vi "Faults_To_String_Array.vi"(0 "Write Header ?":bool, 1 "Fault Table Entry":T1[](array[typedef]), 5 "Error In":errorcluster) -> (15 "Fault Header String Array":string[](array[string]), 16 "Fault ERD Number String Array":string[](array[string]), 17 "Fault Data String Array":string[](array[string]), 19 "Error Out":errorcluster)   [LabVIEW 2023]
uses:
  type defs/Fault_Table_Info.ctl
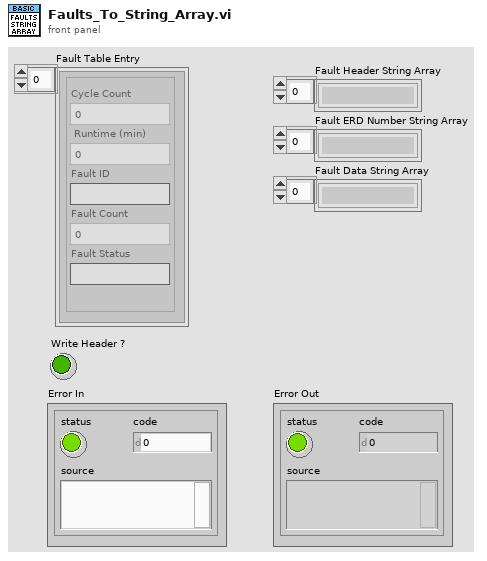
[diagram p1: front panel]
types:
  T1 = typedef "Fault_Table_Info.ctl" = cluster{"Cycle Count":u32, " Runtime (min) ":u32, "Fault Status":string, "Fault ID":string, "Fault Count":u16}
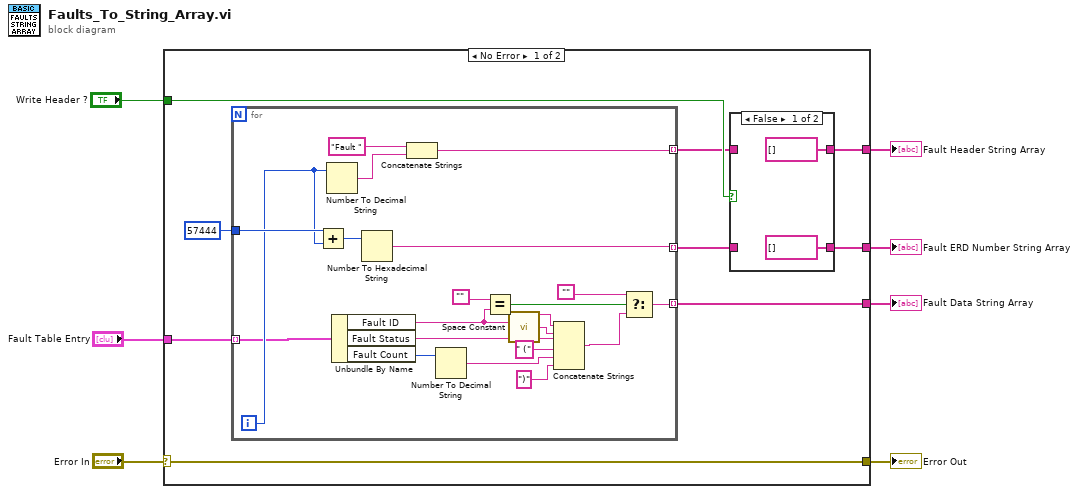
[diagram p0: block diagram]
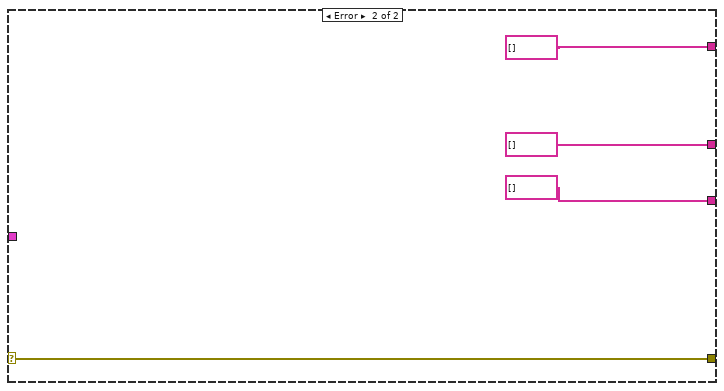
[diagram p3: hidden frame]
diagram:
  n1 = case shown="No Error" "Error In" {
    selector: "Error In" -> [w14 w43]
    tunnel: "Fault Table Entry" -> [w16 _]
    tunnel: [w15 string[] []] -> w6
    tunnel: [w14 w43] -> w4
    tunnel: [w10 string[] []] -> w3
    tunnel: [w8 string[] []] -> w2
    tunnel: "Write Header ?" -> [w12 _]
    frame No Error {
      n2 = for {
        tunnel: [w33] -> w15 mode=indexing
        tunnel: w16 -> [w27] mode=indexing
        tunnel: [w31] -> w11 mode=indexing
        tunnel: 57444 -> [w30]
        tunnel: [w28] -> w9 mode=indexing
        i -> [w29]
        n3 = Add(x=w30, y=w29) -> (x+y=w21:i32)
        n4 = Number To Decimal String(number=w29) -> (decimal integer string=w22:string)  [unwired: 1 in]
        n5 = Unbundle By Name(w27) -> ("Fault ID"=w26:string, "Fault Status"=w25:string, "Fault Count"=w24:u16)
        n6 = Number To Hexadecimal String(2:w21) -> (0:w28:string)  [unwired: 1 in]
        n7 = Concatenate Strings("Fault ", w22) -> (w31:string)
        n8 = Number To Decimal String(number=w24) -> (decimal integer string=w38:string)  [unwired: 1 in]
        n9 = Equal?(x="", y=w26) -> (x = y?=w35:bool)
        n10 = call <vilib>:"Space Constant.vi"() -> ("String"=w40:string)
        n11 = Concatenate Strings(w26, w40, w25, " (" ("string"), w38, ")" ("string")) -> (w34:string)
        n12 = Select(t="", s=w35, f=w34) -> (s? t:f=w33:string)
      }
      n13 = case shown="False" w12 {
        tunnel: w11 -> [_ w20]
        tunnel: [string[] [] w20] -> w10
        tunnel: w9 -> [_ w19]
        tunnel: [string[] [] w19] -> w8
        frame False {
        }
        frame True {
        }
      }
    }
    frame Error {
    }
  }
  "Fault Data String Array" <- w6
  "Error Out" <- w4
  "Fault Header String Array" <- w3
  "Fault ERD Number String Array" <- w2
